vi "prueba2.vi"(11 "IRQ Number":u8) -> ()   [LabVIEW 2017]
uses:
  <vilib>/myRIO/Common/Instrument Driver Framework/myRIO v1.0/myRIO v1.0 Close.vi
  <vilib>/myRIO/Common/Instrument Driver Framework/Utilities/vis/FPGA Ref Manager.vi
  <vilib>/myRIO/Common/Instrument Driver Framework/myRIO v1.0/IRQ/vis/myRIO v1.0 Reserve IRQ.vi
  <vilib>/myRIO/Instrument Drivers/IRQ/IO IRQ/IO IRQ.lvlib
panel:
  out "Stop?":bool
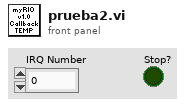
[diagram p1: front panel]
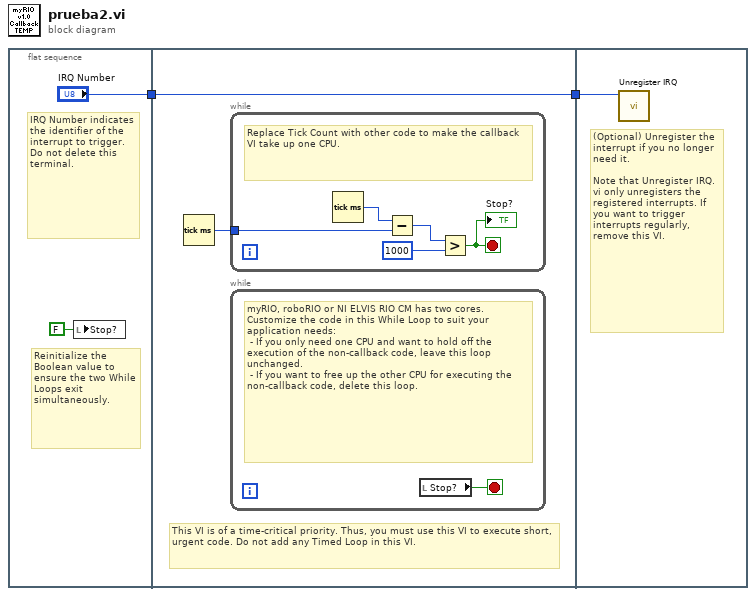
[diagram p0: block diagram]
diagram:
  n1 = flat-sequence {
    tunnel: ["IRQ Number"] -> w2
    tunnel: [w6] -> w1
    tunnel: w2 -> [w6]
    tunnel: w1 -> [w13]
    frame #0 {
      # "Reinitialize the Boolean value to ensure the two While Loops exit simultaneously."
      # "IRQ Number indicates the identifier of the interrupt to trigger. Do not delete this terminal."
      n2 = local write "Stop?"(FALSE ("Stop?")) -> ()
    }
    frame #1 {
      # "This VI is of a time-critical priority. Thus, you must use this VI to execute short, urgent code. Do not add any Timed Loop in this VI."
      n3 = Tick Count (ms)() -> (millisecond timer value=w5:u32)
      n4 = while {
        tunnel: w5 -> [w9]
        stop <- w8 stop-if-true
        # "Replace Tick Count with other code to make the callback VI take up one CPU."
        n5 = Tick Count (ms)() -> (millisecond timer value=w10:u32)
        n6 = Subtract(x=w10, y=w9) -> (x-y=w11:u32)
        n7 = Greater?(x=w11, y=u32 1000) -> (0:w8:bool)
        "Stop?" <- w8
      }
      n8 = while {
        stop <- w7 stop-if-true
        # "myRIO, roboRIO or NI ELVIS RIO CM has two cores. Customize the code in this While Loop to suit your application needs:\n - If you only need one CPU and want to hold off the execution of the non-callback code, leave this loop unchanged.\n - If you want to free up the other CPU for executing the non-callback code, delete this loop."
        n9 = local read "Stop?"() -> (w7:bool)
      }
    }
    frame #2 {
      # "(Optional) Unregister the interrupt if you no longer need it.\n\nNote that Unregister IRQ.vi only unregisters the registered interrupts. If you want to trigger interrupts regularly, remove this VI."
      n10 = call <vilib>:"Unregister IRQ.vi"("IRQ Number"=w13) -> ()  [unwired: 10 in, 1 out]
    }
  }
